vi "32chFFT.vi"(10 "频率":dbl, 11 "32chFFT":T2) -> (2 "频谱图":dbl[](graph), 3 "32value":T1)   [LabVIEW 2014]
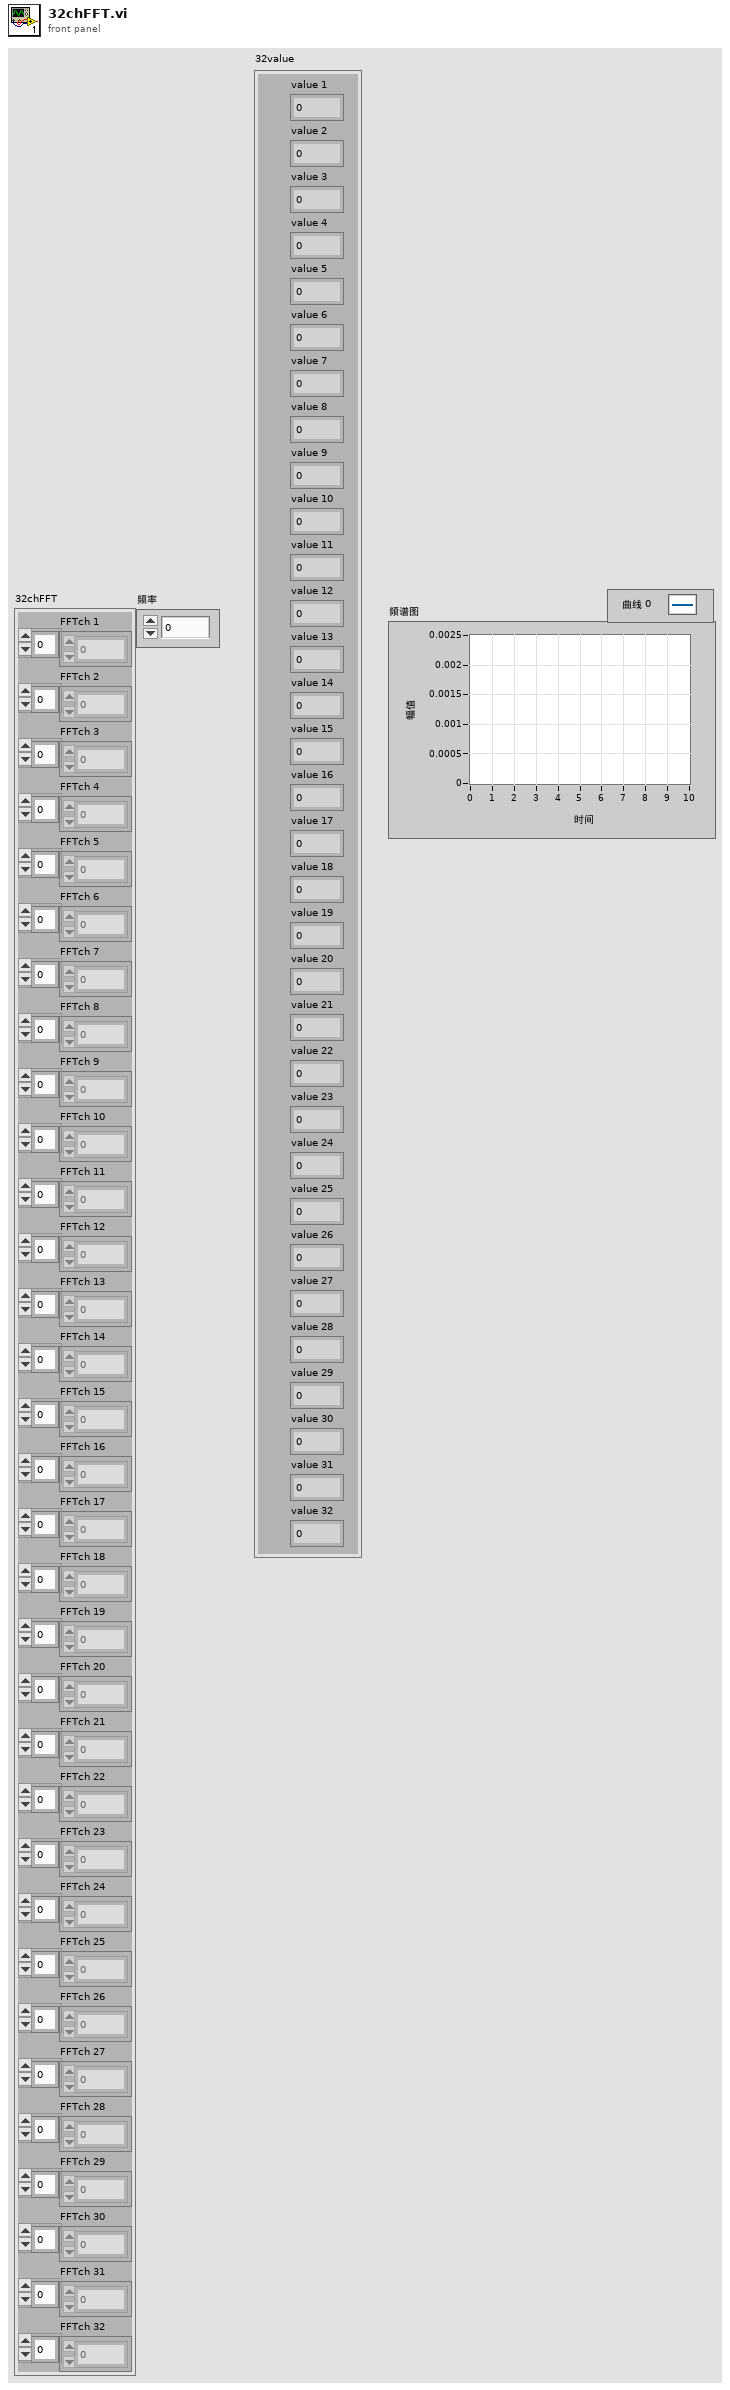
[diagram p1: front panel]
types:
  T1 = cluster{"value 1":dbl, "value 2":dbl, "value 3":dbl, "value 4":dbl, "value 5":dbl, "value 6":dbl, "value 7":dbl, "value 8":dbl, "value 9":dbl, "value 10":dbl, "value 11":dbl, "value 12":dbl, "value 13":dbl, "value 14":dbl, "value 15":dbl, "value 16":dbl, "value 17":dbl, "value 18":dbl, "value 19":dbl, "value 20":dbl, "value 21":dbl, "value 22":dbl, "value 23":dbl, "value 24":dbl, "value 25":dbl, "value 26":dbl, "value 27":dbl, "value 28":dbl, "value 29":dbl, "value 30":dbl, "value 31":dbl, "value 32":dbl}
  T2 = cluster{"FFTch 1":dbl[], "FFTch 2":dbl[], "FFTch 3":dbl[], "FFTch 4":dbl[], "FFTch 5":dbl[], "FFTch 6":dbl[], "FFTch 7":dbl[], "FFTch 8":dbl[], "FFTch 9":dbl[], "FFTch 10":dbl[], "FFTch 11":dbl[], "FFTch 12":dbl[], "FFTch 13":dbl[], "FFTch 14":dbl[], "FFTch 15":dbl[], "FFTch 16":dbl[], "FFTch 17":dbl[], "FFTch 18":dbl[], "FFTch 19":dbl[], "FFTch 20":dbl[], "FFTch 21":dbl[], "FFTch 22":dbl[], "FFTch 23":dbl[], "FFTch 24":dbl[], "FFTch 25":dbl[], "FFTch 26":dbl[], "FFTch 27":dbl[], "FFTch 28":dbl[], "FFTch 29":dbl[], "FFTch 30":dbl[], "FFTch 31":dbl[], "FFTch 32":dbl[]}
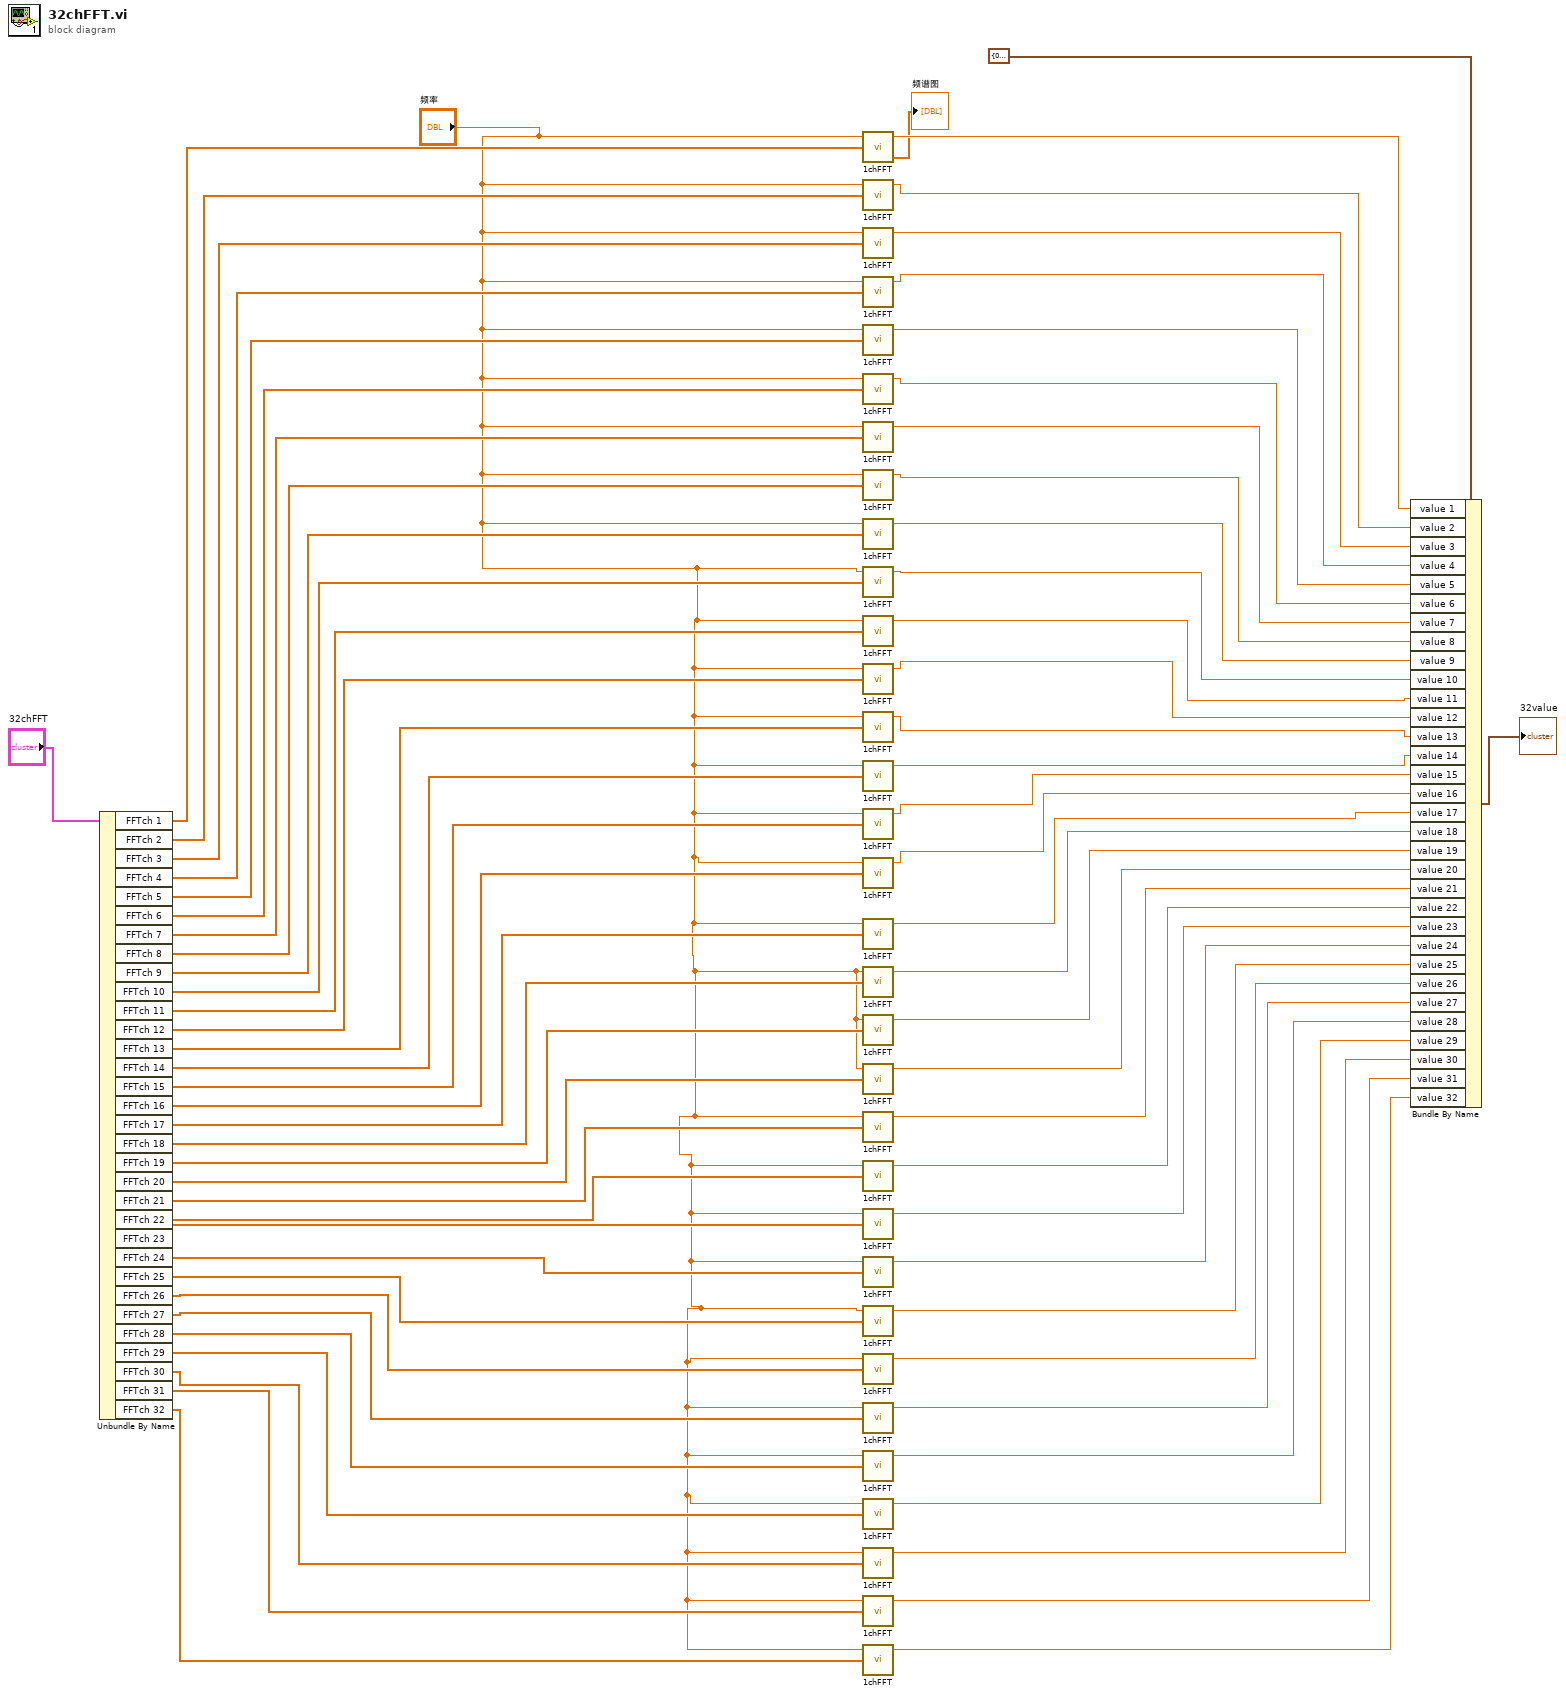
[diagram p0: block diagram]
diagram:
  n1 = Unbundle By Name("32chFFT") -> ("FFTch 1"=w68:dbl[], "FFTch 2"=w67:dbl[], "FFTch 3"=w66:dbl[], "FFTch 4"=w65:dbl[], "FFTch 5"=w64:dbl[], "FFTch 6"=w63:dbl[], "FFTch 7"=w62:dbl[], "FFTch 8"=w61:dbl[], "FFTch 9"=w60:dbl[], "FFTch 10"=w59:dbl[], "FFTch 11"=w58:dbl[], "FFTch 12"=w57:dbl[], "FFTch 13"=w56:dbl[], "FFTch 14"=w55:dbl[], "FFTch 15"=w54:dbl[], "FFTch 16"=w53:dbl[], "FFTch 17"=w52:dbl[], "FFTch 18"=w51:dbl[], "FFTch 19"=w50:dbl[], "FFTch 20"=w49:dbl[], "FFTch 21"=w48:dbl[], "FFTch 22"=w47:dbl[], "FFTch 23"=w46:dbl[], "FFTch 24"=w45:dbl[], "FFTch 25"=w44:dbl[], "FFTch 26"=w43:dbl[], "FFTch 27"=w42:dbl[], "FFTch 28"=w41:dbl[], "FFTch 29"=w40:dbl[], "FFTch 30"=w39:dbl[], "FFTch 31"=w37:dbl[], "FFTch 32"=w38:dbl[])
  n2 = call "1chFFT.vi"("Array"=w68, "频率"="频率") -> ("频谱图"=→"频谱图":dbl[], "幅度值"=w34:dbl)  [unwired: 2 in]
  n3 = call "1chFFT.vi"("Array"=w67, "频率"="频率") -> ("幅度值"=w33:dbl)  [unwired: 2 in, 1 out]
  n4 = call "1chFFT.vi"("Array"=w66, "频率"="频率") -> ("幅度值"=w32:dbl)  [unwired: 2 in, 1 out]
  n5 = call "1chFFT.vi"("Array"=w65, "频率"="频率") -> ("幅度值"=w31:dbl)  [unwired: 2 in, 1 out]
  n6 = call "1chFFT.vi"("Array"=w64, "频率"="频率") -> ("幅度值"=w30:dbl)  [unwired: 2 in, 1 out]
  n7 = call "1chFFT.vi"("Array"=w63, "频率"="频率") -> ("幅度值"=w29:dbl)  [unwired: 2 in, 1 out]
  n8 = call "1chFFT.vi"("Array"=w62, "频率"="频率") -> ("幅度值"=w28:dbl)  [unwired: 2 in, 1 out]
  n9 = call "1chFFT.vi"("Array"=w61, "频率"="频率") -> ("幅度值"=w27:dbl)  [unwired: 2 in, 1 out]
  n10 = call "1chFFT.vi"("Array"=w60, "频率"="频率") -> ("幅度值"=w26:dbl)  [unwired: 2 in, 1 out]
  n11 = call "1chFFT.vi"("Array"=w59, "频率"="频率") -> ("幅度值"=w25:dbl)  [unwired: 2 in, 1 out]
  n12 = call "1chFFT.vi"("Array"=w58, "频率"="频率") -> ("幅度值"=w24:dbl)  [unwired: 2 in, 1 out]
  n13 = call "1chFFT.vi"("Array"=w57, "频率"="频率") -> ("幅度值"=w23:dbl)  [unwired: 2 in, 1 out]
  n14 = call "1chFFT.vi"("Array"=w56, "频率"="频率") -> ("幅度值"=w22:dbl)  [unwired: 2 in, 1 out]
  n15 = call "1chFFT.vi"("Array"=w55, "频率"="频率") -> ("幅度值"=w21:dbl)  [unwired: 2 in, 1 out]
  n16 = call "1chFFT.vi"("Array"=w54, "频率"="频率") -> ("幅度值"=w20:dbl)  [unwired: 2 in, 1 out]
  n17 = call "1chFFT.vi"("Array"=w53, "频率"="频率") -> ("幅度值"=w19:dbl)  [unwired: 2 in, 1 out]
  n18 = call "1chFFT.vi"("Array"=w52, "频率"="频率") -> ("幅度值"=w18:dbl)  [unwired: 2 in, 1 out]
  n19 = call "1chFFT.vi"("Array"=w51, "频率"="频率") -> ("幅度值"=w17:dbl)  [unwired: 2 in, 1 out]
  n20 = call "1chFFT.vi"("Array"=w50, "频率"="频率") -> ("幅度值"=w16:dbl)  [unwired: 2 in, 1 out]
  n21 = call "1chFFT.vi"("Array"=w49, "频率"="频率") -> ("幅度值"=w15:dbl)  [unwired: 2 in, 1 out]
  n22 = call "1chFFT.vi"("Array"=w48, "频率"="频率") -> ("幅度值"=w14:dbl)  [unwired: 2 in, 1 out]
  n23 = call "1chFFT.vi"("Array"=w47, "频率"="频率") -> ("幅度值"=w13:dbl)  [unwired: 2 in, 1 out]
  n24 = call "1chFFT.vi"("Array"=w46, "频率"="频率") -> ("幅度值"=w12:dbl)  [unwired: 2 in, 1 out]
  n25 = call "1chFFT.vi"("Array"=w45, "频率"="频率") -> ("幅度值"=w11:dbl)  [unwired: 2 in, 1 out]
  n26 = call "1chFFT.vi"("Array"=w44, "频率"="频率") -> ("幅度值"=w10:dbl)  [unwired: 2 in, 1 out]
  n27 = call "1chFFT.vi"("Array"=w43, "频率"="频率") -> ("幅度值"=w9:dbl)  [unwired: 2 in, 1 out]
  n28 = call "1chFFT.vi"("Array"=w42, "频率"="频率") -> ("幅度值"=w8:dbl)  [unwired: 2 in, 1 out]
  n29 = call "1chFFT.vi"("Array"=w41, "频率"="频率") -> ("幅度值"=w7:dbl)  [unwired: 2 in, 1 out]
  n30 = call "1chFFT.vi"("Array"=w40, "频率"="频率") -> ("幅度值"=w6:dbl)  [unwired: 2 in, 1 out]
  n31 = call "1chFFT.vi"("Array"=w39, "频率"="频率") -> ("幅度值"=w5:dbl)  [unwired: 2 in, 1 out]
  n32 = call "1chFFT.vi"("Array"=w37, "频率"="频率") -> ("幅度值"=w4:dbl)  [unwired: 2 in, 1 out]
  n33 = call "1chFFT.vi"("Array"=w38, "频率"="频率") -> ("幅度值"=w3:dbl)  [unwired: 2 in, 1 out]
  n34 = Bundle By Name(cluster=T1 {"value 1"=0.0, "value 2"=0.0, "value 3"=0.0, "value 4"=0.0, "value 5"=0.0, "value 6"=0.0, "value 7"=0.0, "value 8"=0.0, "value 9"=0.0, "value 10"=0.0, "value 11"=0.0, "value 12"=0.0, "value 13"=0.0, "value 14"=0.0, "value 15"=0.0, "value 16"=0.0, "value 17"=0.0, "value 18"=0.0, "value 19"=0.0, "value 20"=0.0, "value 21"=0.0, "value 22"=0.0, "value 23"=0.0, "value 24"=0.0, "value 25"=0.0, "value 26"=0.0, "value 27"=0.0, "value 28"=0.0, "value 29"=0.0, "value 30"=0.0, "value 31"=0.0, "value 32"=0.0} ("32value"), "value 1"=w34, "value 2"=w33, "value 3"=w32, "value 4"=w31, "value 5"=w30, "value 6"=w29, "value 7"=w28, "value 8"=w27, "value 9"=w26, "value 10"=w25, "value 11"=w24, "value 12"=w23, "value 13"=w22, "value 14"=w21, "value 15"=w20, "value 16"=w19, "value 17"=w18, "value 18"=w17, "value 19"=w16, "value 20"=w15, "value 21"=w14, "value 22"=w13, "value 23"=w12, "value 24"=w11, "value 25"=w10, "value 26"=w9, "value 27"=w8, "value 28"=w7, "value 29"=w6, "value 30"=w5, "value 31"=w4, "value 32"=w3) -> (→"32value":T1)
